vi "Read TEC Data.vi"(8 "error in":errorcluster, 11 "CRDS Data in":refnum<class "CRDS Data.lvclass">) -> (0 "error out":errorcluster, 2 "tecData":cluster{"T":dbl, "Power":dbl}, 3 "CRDS Data out":refnum<class "CRDS Data.lvclass">)   [LabVIEW 2011, in "CRDS Data.lvclass"]
uses:
  CRDS Data.lvclass
  Reusable/DataClass/TECooler/TECData.lvclass
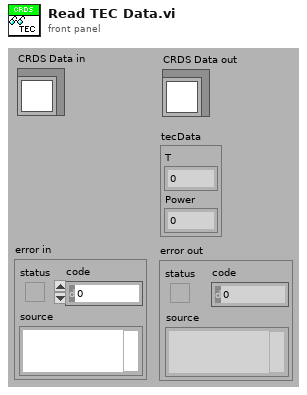
[diagram p1: front panel]
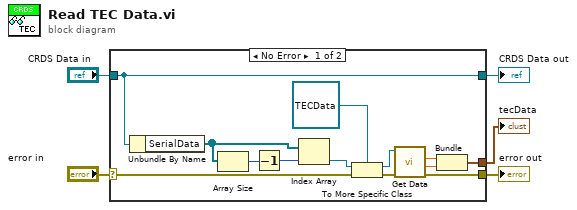
[diagram p0: block diagram]
diagram:
  n1 = case shown="No Error" "error in" {
    selector: "error in" -> [w12 w20]
    tunnel: [w7 w20] -> w4
    tunnel: [w18 w19] -> w2
    tunnel: "CRDS Data in" -> [w18 w19]
    tunnel: [w6 _] -> w1
    frame No Error {
      n2 = Unbundle By Name(w18) -> ("SerialData"=w15:refnum<class "Data.lvclass">[])
      n3 = Array Size(array=w15) -> (size(s)=w17:i32)
      n4 = Decrement(x=w17) -> (x-1=w16:i32)
      n5 = Index Array(array=w15, index=w16) -> (element=w13:refnum<class "Data.lvclass">)
      n6 = To More Specific Class(target class=refnum<class "TECData.lvclass"> refnum ("TECData.lvclass"), reference=w13, error in=w12) -> (specific class reference=w11:refnum<class "TECData.lvclass">, error out=w10:errorcluster)
      n7 = call "Get Data.vi"("error in (no error)"=w10, "TECData in"=w11) -> ("error out"=w7:errorcluster, "Power"=w8:sgl, "T"=w9:sgl)  [unwired: 6 in, 1 out]
      n8 = Bundle("T"=w9, "Power"=w8) -> (w6:cluster{"T":sgl, "Power":sgl})  [unwired: 1 in]
    }
    frame Error {
    }
  }
  "error out" <- w4
  "CRDS Data out" <- w2
  "tecData" <- w1
